vi "ex12-1.vi"() -> ()   [LabVIEW 2009]
uses:
  <vilib>/NXT/Subs/LVHSConnector.ctl
  <vilib>/NXT/Block Support/NXT_InputPort.ctl
  mindsensors.com LVEE Toolkit/Dual/NXTLineLeader-DM.vi
  mindsensors.com LVEE Toolkit/Dual/NXTLineLeader-Util-DM.vi
  <vilib>/NXT/Subs/MotorOutput.ctl
panel:
  out "Output of NXTLineLeader":T1={"Average"=247, "Steering"=0, "Base Direction"=FALSE, "Base Power"=50, "Motor 1 Direction"=FALSE, "Motor 1 Power"=55, "Motor 2 Direction"=FALSE, "Motor 2 Power"=45, "Success?"=TRUE}
  in  "Input of NXTLineLeader-Util":T2={"Kp"=25, "Ki"=0, "Kd"=15, "SetPoint"=45, "Kp_factor"=32, "Ki_factor"=32, "Kd_factor"=32} {"Kd_factor" min=1; "Ki_factor" min=1; "Kp_factor" min=1; "SetPoint" max=80}
  in  "Input of NXTLineLeader":T3={"Base Power"=50, "Base Direction"=FALSE, "Operation"=enum."Track Line"} {"Base Power" min=0 max=100}
  in  "Input Port":T4 items=["Port 1", "Port 2", "Port 3", "Port 4"]
  in  "Base Direction":string="BCKWRD"
  in  "MD2":string="BCKWRD"
  in  "MD1":string="BCKWRD"
  out "NXT dup":T5={"error"={"status"=FALSE, "code"=0, "source"=""}, "address"="USB0::0x0694::0x0002::0016530DBBF2::RAW", "NXT #"=0, "Show Error"=FALSE, "Connection"=4} {"Connection" items=["USB", "Bluetooth", "USB then Bluetooth", "Last Connection", "Preference"]}
  in  "NXT":T5={"error"={"status"=FALSE, "code"=0, "source"=""}, "address"="", "NXT #"=-1, "Show Error"=TRUE, "Connection"=4} {"Connection" items=["USB", "Bluetooth", "USB then Bluetooth", "Last Connection", "Preference"]}
  in  "?":bool
  # "mindsensors.com\nCopyright (c) 2009 by mindsensors.com\nEmail: info (<at>) mindsensors (<dot>) com\n\nThis program is free software. You can redistribute it and/or modify\nit under the terms of the GNU General Public License as published by\nthe Free Software Foundation; version 3 of the License.\nRead the license at: http://www.gnu.org/licenses/gpl.txt"
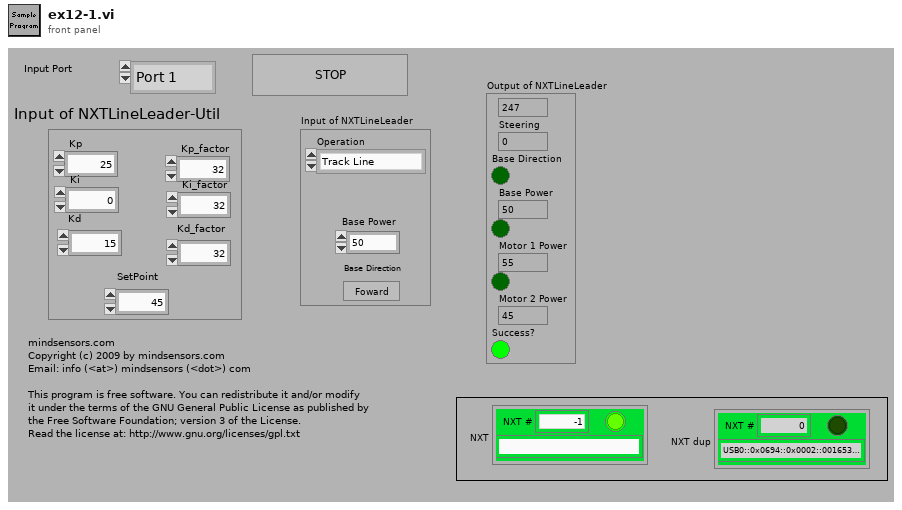
[diagram p1: front panel]
types:
  T1 = cluster{"Average":u8, "Steering":i8, "Base Direction":bool, "Base Power":i8, "Motor 1 Direction":bool, "Motor 1 Power":i32, "Motor 2 Direction":bool, "Motor 2 Power":i32, "Success?":bool}
  T2 = cluster{"Kp":u8, "Ki":u8, "Kd":u8, "SetPoint":u8, "Kp_factor":u8, "Ki_factor":u8, "Kd_factor":u8}
  T3 = cluster{"Base Power":i8, "Base Direction":bool, "Operation":enum32{"Track Line", "Read Raw Sensor ", "Read Sensor Avg"}}
  T4 = typedef "NXT_InputPort.ctl" = u8
  T5 = typedef "LVHSConnector.ctl" = cluster{"error":errorcluster, "address":string, "NXT #":i32, "Show Error":bool, "Connection":u16}
  T6 = typedef "MotorOutput.ctl" = u8
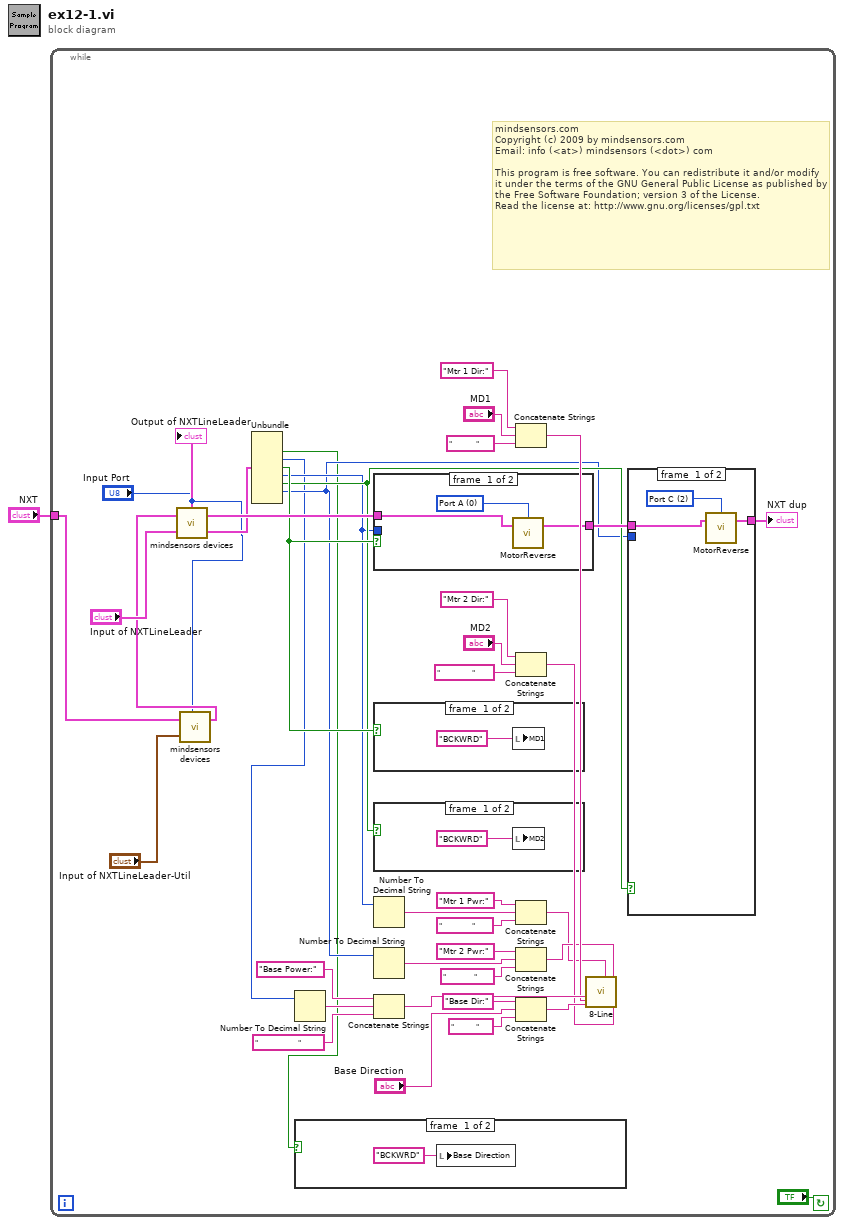
[diagram p0: block diagram]
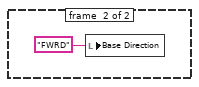
[diagram p2: hidden frame]
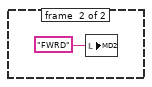
[diagram p3: hidden frame]
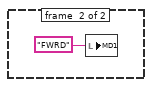
[diagram p4: hidden frame]
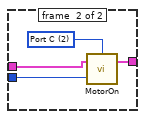
[diagram p5: hidden frame]
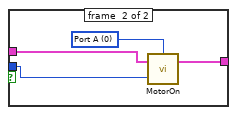
[diagram p6: hidden frame]
diagram:
  n1 = while {
    tunnel: "NXT" -> [w9]
    stop <- "?" continue-if-true
    # "mindsensors.com\nCopyright (c) 2009 by mindsensors.com\nEmail: info (<at>) mindsensors (<dot>) com\n\nThis program is free software. You can redistribute it and/or modify\nit under the terms of the GNU General Public License as published by\nthe Free Software Foundation; version 3 of the License.\nRead the license at: http://www.gnu.org/licenses/gpl.txt"
    n2 = call-poly "mindsensors devices.vi"("Input of NXTLineLeader-Util"="Input of NXTLineLeader-Util", "NXT"=w9, "Input Port"="Input Port") -> ("NXT dup"=w10:T5)  [unwired: 1 out]
    n3 = call-poly "mindsensors devices.vi"("Input of NXTLineLeader"="Input of NXTLineLeader", "NXT"=w10, "Input Port"="Input Port") -> ("Output of NXTLineLeader"=w13:T1, "NXT dup"=w40:T5)
    "Output of NXTLineLeader" <- w13
    n4 = Unbundle(w13) -> ("Base Direction"=w2:bool, "Base Power"=w3:i8, "Motor 1 Direction"=w7:bool, "Motor 1 Power"=w5:i32, "Motor 2 Direction"=w6:bool, "Motor 2 Power"=w4:i32)  [unwired: 3 out]
    n5 = Number To Decimal String(number=w3) -> (decimal integer string=w35:string)  [unwired: 1 in]
    n6 = case shown="False" w2 {
      frame #0 {
        n7 = local write "Base Direction"("BCKWRD") -> ()
      }
      frame #1 {
        n8 = local write "Base Direction"("FWRD") -> ()
      }
    }
    n9 = case shown="True" w7 {
      tunnel: w40 -> [w57 w61]
      tunnel: [w56 w59] -> w39
      tunnel: w5 -> [_ w58]
      frame #0 {
        w55 = T6 0 items=["Port A", "Port B", "Port C", "All Ports"] ("Output Port")
        n10 = call <vilib>:"MotorReverse.vi"("NXT"=w57, "Output Port (All Ports)"=w55) -> ("NXT"=w56:T5)  [unwired: 2 in]
      }
      frame #1 {
        w60 = T6 0 items=["Port A", "Port B", "Port C", "All Ports"] ("Output Port")
        n11 = call <vilib>:"MotorOn.vi"("Power (75)"=w58, "NXT"=w61, "Output Port (All Ports)"=w60) -> ("NXT"=w59:T5)  [unwired: 1 in]
      }
    }
    n12 = case shown="False" w7 {
      frame #0 {
        n13 = local write "MD1"("BCKWRD") -> ()
      }
      frame #1 {
        n14 = local write "MD1"("FWRD") -> ()
      }
    }
    n15 = case shown="False" w6 {
      frame #0 {
        n16 = local write "MD2"("BCKWRD") -> ()
      }
      frame #1 {
        n17 = local write "MD2"("FWRD") -> ()
      }
    }
    n18 = Number To Decimal String(number=w5) -> (decimal integer string=w20:string)  [unwired: 1 in]
    n19 = Number To Decimal String(number=w4) -> (decimal integer string=w19:string)  [unwired: 1 in]
    n20 = Concatenate Strings("Base Power:" ("string"), w35, "                    " ("string")) -> (w34:string)
    n21 = Concatenate Strings("Mtr 1 Dir:" ("string"), "MD1", "            " ("string")) -> (w24:string)
    n22 = Concatenate Strings("Mtr 2 Dir:" ("string"), "MD2", "                " ("string")) -> (w23:string)
    n23 = Concatenate Strings("Mtr 1 Pwr:" ("string"), w20, "               " ("string")) -> (w15:string)
    n24 = Concatenate Strings("Mtr 2 Pwr:" ("string"), w19, "              " ("string")) -> (w16:string)
    n25 = Concatenate Strings("Base Dir:" ("string"), "Base Direction", "           " ("string")) -> (w31:string)
    n26 = call "8-Line.vi"("Line 7"=w16, "Line 6"=w23, "Line 5"=w15, "Line 4"=w24, "Line 3"=w31, "Line 2"=w34) -> ()  [unwired: 5 in, 1 out]
    n27 = case shown="True" w6 {
      tunnel: w39 -> [w50 w54]
      tunnel: [w49 w52] -> w38
      tunnel: w4 -> [_ w51]
      frame #0 {
        w48 = T6 2 items=["Port A", "Port B", "Port C", "All Ports"] ("Output Port")
        n28 = call <vilib>:"MotorReverse.vi"("NXT"=w50, "Output Port (All Ports)"=w48) -> ("NXT"=w49:T5)  [unwired: 2 in]
      }
      frame #1 {
        w53 = T6 2 items=["Port A", "Port B", "Port C", "All Ports"] ("Output Port")
        n29 = call <vilib>:"MotorOn.vi"("Power (75)"=w51, "NXT"=w54, "Output Port (All Ports)"=w53) -> ("NXT"=w52:T5)  [unwired: 1 in]
      }
    }
    "NXT dup" <- w38
  }
